vi "setUp.vi"(8 "error in (no error)":errorcluster, 11 "reference in":refnum<class "Instrument Addon System Tests.lvclass">) -> (0 "error out":errorcluster, 3 "reference out":refnum<class "Instrument Addon System Tests.lvclass">)   [LabVIEW 2019, in "Instrument Addon System Tests.lvclass"]
doc: "setUp runs prior to the test method during test execution. Use this method to initialize any object data required by your tests."
uses:
  Instrument Addon System Tests.lvclass
  C:/Program Files (x86)/National Instruments/LabVIEW 2019/vi.lib/addons/_JKI Toolkits/VI Tester/TestCase.llb/TestCase.lvclass
  <vilib>/addons/_JKI Toolkits/VI Tester/TestCase.llb/TestCase.lvclass
  C:/Dev/ni-master/niveristand-custom-device-testing-tools/VeriStandTestCase/VeriStandTestCase.lvclass
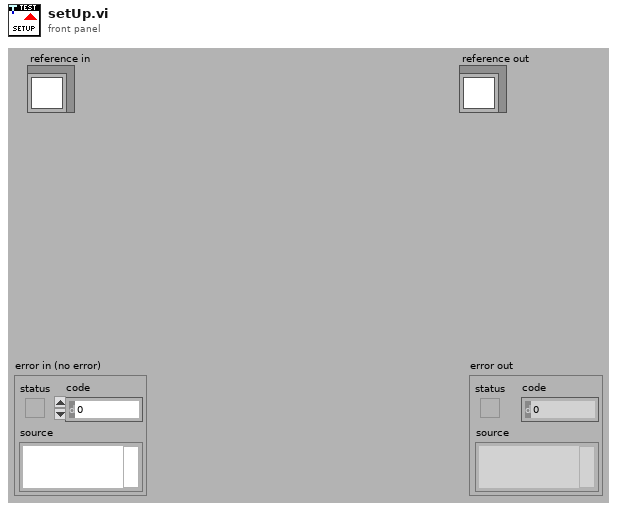
[diagram p1: front panel]
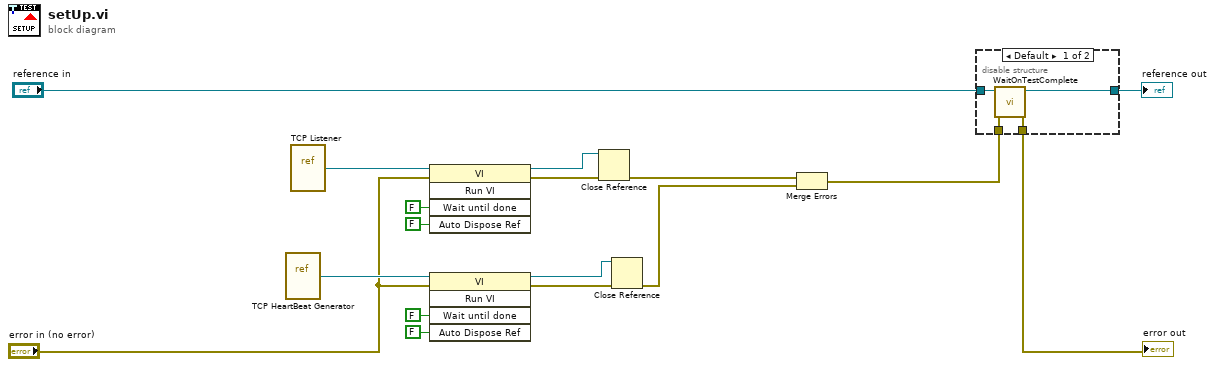
[diagram p0: block diagram]
diagram:
  n1 = vi-ref "TCP HeartBeat Generator.vi"() -> (w6:refnum<vi>)
  n2 = vi-ref "TCP Listener.vi"() -> (w14:refnum<vi>)
  n3 = invoke class="VI" method="Run VI"(reference=w14, error in="error in (no error)", "Wait until done"=FALSE ("Wait Until Done"), "Auto Dispose Ref"=FALSE ("Auto Dispose Reference")) -> (reference out=w13:refnum<vi>, error out=w12:errorcluster)  [unwired: 1 in, 3 out]
  n4 = invoke class="VI" method="Run VI"(reference=w6, error in="error in (no error)", "Wait until done"=FALSE ("Wait Until Done"), "Auto Dispose Ref"=FALSE ("Auto Dispose Reference")) -> (reference out=w3:refnum<vi>, error out=w2:errorcluster)  [unwired: 1 in, 3 out]
  n5 = Close Reference(reference=w13, error in (no error)=w12) -> (error out=w11:errorcluster)
  n6 = Close Reference(reference=w3, error in (no error)=w2) -> (error out=w1:errorcluster)
  n7 = Merge Errors(w11, w1) -> (w8:errorcluster)
  n8 = disable-structure shown="Default" {
    disable-tunnel: w8 -> [w21 w22]
    disable-tunnel: [w20 w22] -> w17
    disable-tunnel: [w19 w23] -> w16
    disable-tunnel: "reference in" -> [w18 w23]
    frame condition #0 (active) {
      n9 = call <vilib>:"WaitOnTestComplete.vi"("error in (no error)"=w21, "TestCase in"=w18) -> ("error out"=w20:errorcluster, "TestCase in"=w19:refnum<class "Instrument Addon System Tests.lvclass">)  [unwired: 8 in]
    }
    frame condition #1 {
    }
  }
  "error out" <- w17
  "reference out" <- w16
